vi "Uniform Random.vi"(6 "seed":i32=-1, 7 "reset":bool, 9 "xmax":dbl=1.0, 10 "xmin":dbl, 11 "samples":i32=128) -> (0 "error":i32, 3 "uniform random data":dbl[](array[numeric]))   [LabVIEW 2014, in "NI_Gmath.lvlib"]
doc: "Generates random values from a variate X, where X describes the selected distribution type. You must manually select the polymorphic instance to use."
uses:
  NI_Gmath.lvlib
  NI_AALBase.lvlib
panel:
  # "Uniform Random"
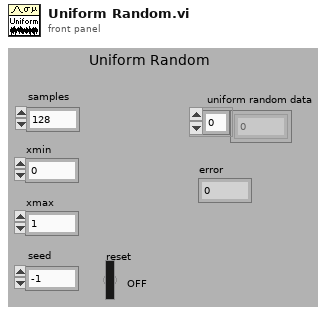
[diagram p1: front panel]
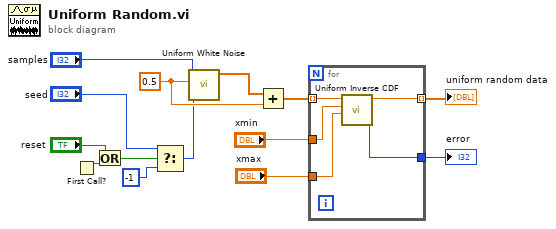
[diagram p0: block diagram]
diagram:
  w12 = 0.5 ("amplitude")
  n1 = First Call?() -> (First Call?: T/F=w6:bool)
  n2 = Or(x="reset", y=w6) -> (x .or. y?=w5:bool)
  n3 = Select(t="seed", s=w5, f=-1) -> (s? t:f=w1:i32)
  n4 = call "Uniform White Noise.vi"("seed"=w1, "amplitude"=w12, "samples"="samples") -> ("uniform white noise"=w13:dbl[])  [unwired: 7 in, 1 out]
  n5 = Add(x=w13, y=w12) -> (x+y=w11:dbl[])
  n6 = for {
    tunnel: w11 -> [w19] mode=indexing
    tunnel: "xmin" -> [w18]
    tunnel: "xmax" -> [w17]
    tunnel: [w16] -> w8 mode=indexing
    tunnel: [w15] -> w7
    n7 = call "Uniform Inverse CDF.vi"("xmax"=w17, "xmin"=w18, "cdf(x)"=w19) -> ("error"=w15:i32, "x"=w16:dbl)  [unwired: 7 in]
  }
  "error" <- w7
  "uniform random data" <- w8
